vi "glyph_pass.vi"() -> (1 "image data":T1={"image type"=0, "image depth"=32, "image"=[0, 0, 0, 0, 0, 0, 0, 0, 0, 0, 0, 0, 0, 0, 0, 0, 0, 0, 0, 0, 255, 0, 0, 0, 255, 0, 0, 0, 255, 0, 0, 0, 255, 0, 0, 0, 255, 0, 0, 0, 0, 0, 0, 0, 0, 0, 0, 0, 0, 0, 0, 0, 0, 0, 0, 0, 0, 0, 0, 0, 0, 0, 0, 0, 0, 0, 0, 0, 0, 0, 0, 0, 0, 0, 0, 0, 255, 0, 0, 0, 255, 0, 0, 0, 255, 0, 255, 0, 255, 0, 255, 0, 255, 0, 255, 0, 255, 0, 255, 0, 255, 0, 255, 0, 255, 0, 0, 0, 255, 0, 0, 0, 0, 0, 0, 0, 0, 0, 0, 0, 0, 0, 0, 0, 0, 0, 0, 0, 0, 0, 0, 0, 0, 0, 0, 0, 255, 0, 0, 0, 255, 0, 255, 0, 255, 0, 255, 0, 255, 0, 128, 0, 255, 0, 128, 0, 255, 0, 128, 0, 255, 0, 128, 0, 255, 0, 128, 0, 255, 0, 128, 0, 255, 0, 128, 0, 255, 0, 0, 0, 0, 0, 0, 0, 0, 0, 0, 0, 0, 0, 0, 0, 0, 0, 0, 0, 255, 0, 0, 0, 255, 0, 255, 0, 255, 0, 128, 0, 255, 0, 128, 0, 255, 0, 128, 0, 255, 0, 128, 0, 255, 0, 128, 0, 255, 0, 128, 0, 255, 0, 128, 0, 255, 0, 128, 0, 255, 0, 128, 0, 255, 0, 128, 0, 255, 0, 0, 0, 0, 0, 0, 0, 0, 0, 0, 0, 0, 0, 0, 0, 255, 0, 0, 0, 255, 0, 255, 0, 255, 0, 128, 0, 255, 0, 128, 0, 255, 0, 128, 0, 255, 0, 128, 0, 255, 0, 128, 0, 255, 0, 128, 0, 255, 0, 128, 0, 255, 255, 255, 255, 255, 0, 128, 0, 255, 0, 128, 0, 255, 0, 0, 0, 0, 0, 0, 0, 0, 0, 0, 0, 255, 0, 0, 0, 255, 0, 255, 0, 255, 0, 128, 0, 255, 0, 128, 0, 255, 0, 128, 0, 255, 0, 128, 0, 255, 0, 128, 0, 255, 0, 128, 0, 255, 0, 128, 0, 255, 255, 255, 255, 255, 255, 255, 255, 255, 0, 128, 0, 255, 0, 128, 0, 255, 0, 128, 0, 255, 0, 0, 0, 0, 0, 0, 0, 255, 0, 0, 0, 255, 0, 255, 0, 255, 0, 128, 0, 255, 0, 128, 0, 255, 255, 255, 255, 255, 0, 128, 0, 255, 0, 128, 0, 255, 0, 128, 0, 255, 255, 255, 255, 255, 255, 255, 255, 255, 255, 255, 255, 255, 0, 128, 0, 255, 0, 128, 0, 255, 0, 128, 0, 255, 0, 0, 0, 255, 128, 128, 128, 255, 0, 0, 0, 255, 0, 255, 0, 255, 0, 128, 0, 255, 0, 128, 0, 255, 255, 255, 255, 255, 255, 255, 255, 255, 0, 128, 0, 255, 255, 255, 255, 255, 255, 255, 255, 255, 255, 255, 255, 255, 0, 128, 0, 255, 0, 128, 0, 255, 0, 128, 0, 255, 0, 128, 0, 255, 0, 0, 0, 255, 128, 128, 128, 255, 0, 0, 0, 255, 0, 255, 0, 255, 0, 128, 0, 255, 0, 128, 0, 255, 255, 255, 255, 255, 255, 255, 255, 255, 255, 255, 255, 255, 255, 255, 255, 255, 255, 255, 255, 255, 0, 128, 0, 255, 0, 128, 0, 255, 0, 128, 0, 255, 0, 128, 0, 255, 0, 128, 0, 255, 0, 0, 0, 255, 128, 128, 128, 255, 0, 0, 0, 255, 0, 255, 0, 255, 0, 128, 0, 255, 0, 128, 0, 255, 0, 128, 0, 255, 255, 255, 255, 255, 255, 255, 255, 255, 255, 255, 255, 255, 0, 128, 0, 255, 0, 128, 0, 255, 0, 128, 0, 255, 0, 128, 0, 255, 0, 128, 0, 255, 0, 128, 0, 255, 0, 0, 0, 255, 128, 128, 128, 0, 0, 0, 0, 255, 0, 0, 0, 255, 0, 255, 0, 255, 0, 128, 0, 255, 0, 128, 0, 255, 0, 128, 0, 255, 255, 255, 255, 255, 0, 128, 0, 255, 0, 128, 0, 255, 0, 128, 0, 255, 0, 128, 0, 255, 0, 128, 0, 255, 0, 128, 0, 255, 0, 0, 0, 255, 132, 132, 132, 255, 128, 128, 128, 0, 0, 0, 0, 255, 0, 0, 0, 255, 0, 255, 0, 255, 0, 128, 0, 255, 0, 128, 0, 255, 0, 128, 0, 255, 0, 128, 0, 255, 0, 128, 0, 255, 0, 128, 0, 255, 0, 128, 0, 255, 0, 128, 0, 255, 0, 128, 0, 255, 0, 128, 0, 255, 0, 0, 0, 255, 132, 132, 132, 255, 128, 128, 128, 0, 0, 0, 0, 0, 0, 0, 0, 255, 0, 0, 0, 255, 0, 128, 0, 255, 0, 128, 0, 255, 0, 128, 0, 255, 0, 128, 0, 255, 0, 128, 0, 255, 0, 128, 0, 255, 0, 128, 0, 255, 0, 128, 0, 255, 0, 128, 0, 255, 0, 0, 0, 255, 132, 132, 132, 255, 128, 128, 128, 0, 0, 0, 0, 0, 0, 0, 0, 0, 0, 0, 0, 0, 0, 0, 0, 255, 0, 0, 0, 255, 0, 0, 0, 255, 0, 128, 0, 255, 0, 128, 0, 255, 0, 128, 0, 255, 0, 128, 0, 255, 0, 128, 0, 255, 0, 0, 0, 255, 0, 0, 0, 255, 132, 132, 132, 255, 128, 128, 128, 0, 0, 0, 0, 0, 0, 0, 0, 0, 0, 0, 0, 0, 0, 0, 0, 0, 0, 0, 0, 0, 0, 0, 0, 0, 0, 0, 0, 255, 0, 0, 0, 255, 0, 0, 0, 255, 0, 0, 0, 255, 0, 0, 0, 255, 0, 0, 0, 255, 132, 132, 132, 255, 128, 128, 128, 255, 128, 128, 128, 0, 0, 0, 0, 0, 0, 0, 0, 0, 0, 0, 0, 0, 0, 0, 0, 0, 0, 0, 0, 0, 0, 0, 0, 0, 0, 0, 0, 0, 0, 0, 0, 0, 0, 0, 0, 255, 128, 128, 128, 255, 128, 128, 128, 255, 128, 128, 128, 255, 128, 128, 128, 255, 128, 128, 128, 0, 0, 0, 0, 0, 0, 0, 0, 0, 0, 0, 0, 0, 0, 0, 0, 0, 0, 0, 0], "mask"=[7, 192, 31, 240, 63, 248, 127, 252, 127, 252, 255, 254, 255, 255, 255, 255, 255, 255, 255, 255, 127, 255, 127, 255, 63, 254, 31, 252, 7, 248, 3, 224], "colors"=[], "Rectangle"={"left"=0, "top"=0, "right"=16, "bottom"=16}})   [LabVIEW 2015]
uses:
  <vilib>/picture/picture.llb/imagedata.ctl
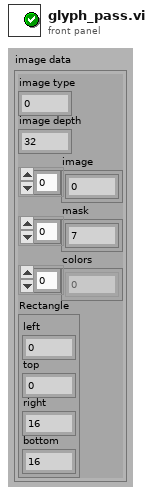
[diagram p1: front panel]
types:
  T1 = typedef "imagedata.ctl" = cluster{"image type":i32, "image depth":i32, "image":u8[], "mask":u8[], "colors":u32[], "Rectangle":cluster{"left":i16, "top":i16, "right":i16, "bottom":i16}}
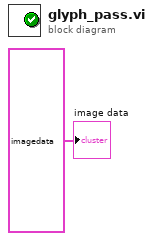
[diagram p0: block diagram]
diagram:
  "image data" <- T1 {"image type"=0, "image depth"=32, "image"=[0, 0, 0, 0, 0, 0, 0, 0, 0, 0, 0, 0, 0, 0, 0, 0, 0, 0, 0, 0, 255, 0, 0, 0, 255, 0, 0, 0, 255, 0, 0, 0, 255, 0, 0, 0, 255, 0, 0, 0, 0, 0, 0, 0, 0, 0, 0, 0, 0, 0, 0, 0, 0, 0, 0, 0, 0, 0, 0, 0, 0, 0, 0, 0, 0, 0, 0, 0, 0, 0, 0, 0, 0, 0, 0, 0, 255, 0, 0, 0, 255, 0, 0, 0, 255, 0, 255, 0, 255, 0, 255, 0, 255, 0, 255, 0, 255, 0, 255, 0, 255, 0, 255, 0, 255, 0, 0, 0, 255, 0, 0, 0, 0, 0, 0, 0, 0, 0, 0, 0, 0, 0, 0, 0, 0, 0, 0, 0, 0, 0, 0, 0, 0, 0, 0, 0, 255, 0, 0, 0, 255, 0, 255, 0, 255, 0, 255, 0, 255, 0, 128, 0, 255, 0, 128, 0, 255, 0, 128, 0, 255, 0, 128, 0, 255, 0, 128, 0, 255, 0, 128, 0, 255, 0, 128, 0, 255, 0, 0, 0, 0, 0, 0, 0, 0, 0, 0, 0, 0, 0, 0, 0, 0, 0, 0, 0, 255, 0, 0, 0, 255, 0, 255, 0, 255, 0, 128, 0, 255, 0, 128, 0, 255, 0, 128, 0, 255, 0, 128, 0, 255, 0, 128, 0, 255, 0, 128, 0, 255, 0, 128, 0, 255, 0, 128, 0, 255, 0, 128, 0, 255, 0, 128, 0, 255, 0, 0, 0, 0, 0, 0, 0, 0, 0, 0, 0, 0, 0, 0, 0, 255, 0, 0, 0, 255, 0, 255, 0, 255, 0, 128, 0, 255, 0, 128, 0, 255, 0, 128, 0, 255, 0, 128, 0, 255, 0, 128, 0, 255, 0, 128, 0, 255, 0, 128, 0, 255, 255, 255, 255, 255, 0, 128, 0, 255, 0, 128, 0, 255, 0, 0, 0, 0, 0, 0, 0, 0, 0, 0, 0, 255, 0, 0, 0, 255, 0, 255, 0, 255, 0, 128, 0, 255, 0, 128, 0, 255, 0, 128, 0, 255, 0, 128, 0, 255, 0, 128, 0, 255, 0, 128, 0, 255, 0, 128, 0, 255, 255, 255, 255, 255, 255, 255, 255, 255, 0, 128, 0, 255, 0, 128, 0, 255, 0, 128, 0, 255, 0, 0, 0, 0, 0, 0, 0, 255, 0, 0, 0, 255, 0, 255, 0, 255, 0, 128, 0, 255, 0, 128, 0, 255, 255, 255, 255, 255, 0, 128, 0, 255, 0, 128, 0, 255, 0, 128, 0, 255, 255, 255, 255, 255, 255, 255, 255, 255, 255, 255, 255, 255, 0, 128, 0, 255, 0, 128, 0, 255, 0, 128, 0, 255, 0, 0, 0, 255, 128, 128, 128, 255, 0, 0, 0, 255, 0, 255, 0, 255, 0, 128, 0, 255, 0, 128, 0, 255, 255, 255, 255, 255, 255, 255, 255, 255, 0, 128, 0, 255, 255, 255, 255, 255, 255, 255, 255, 255, 255, 255, 255, 255, 0, 128, 0, 255, 0, 128, 0, 255, 0, 128, 0, 255, 0, 128, 0, 255, 0, 0, 0, 255, 128, 128, 128, 255, 0, 0, 0, 255, 0, 255, 0, 255, 0, 128, 0, 255, 0, 128, 0, 255, 255, 255, 255, 255, 255, 255, 255, 255, 255, 255, 255, 255, 255, 255, 255, 255, 255, 255, 255, 255, 0, 128, 0, 255, 0, 128, 0, 255, 0, 128, 0, 255, 0, 128, 0, 255, 0, 128, 0, 255, 0, 0, 0, 255, 128, 128, 128, 255, 0, 0, 0, 255, 0, 255, 0, 255, 0, 128, 0, 255, 0, 128, 0, 255, 0, 128, 0, 255, 255, 255, 255, 255, 255, 255, 255, 255, 255, 255, 255, 255, 0, 128, 0, 255, 0, 128, 0, 255, 0, 128, 0, 255, 0, 128, 0, 255, 0, 128, 0, 255, 0, 128, 0, 255, 0, 0, 0, 255, 128, 128, 128, 0, 0, 0, 0, 255, 0, 0, 0, 255, 0, 255, 0, 255, 0, 128, 0, 255, 0, 128, 0, 255, 0, 128, 0, 255, 255, 255, 255, 255, 0, 128, 0, 255, 0, 128, 0, 255, 0, 128, 0, 255, 0, 128, 0, 255, 0, 128, 0, 255, 0, 128, 0, 255, 0, 0, 0, 255, 132, 132, 132, 255, 128, 128, 128, 0, 0, 0, 0, 255, 0, 0, 0, 255, 0, 255, 0, 255, 0, 128, 0, 255, 0, 128, 0, 255, 0, 128, 0, 255, 0, 128, 0, 255, 0, 128, 0, 255, 0, 128, 0, 255, 0, 128, 0, 255, 0, 128, 0, 255, 0, 128, 0, 255, 0, 128, 0, 255, 0, 0, 0, 255, 132, 132, 132, 255, 128, 128, 128, 0, 0, 0, 0, 0, 0, 0, 0, 255, 0, 0, 0, 255, 0, 128, 0, 255, 0, 128, 0, 255, 0, 128, 0, 255, 0, 128, 0, 255, 0, 128, 0, 255, 0, 128, 0, 255, 0, 128, 0, 255, 0, 128, 0, 255, 0, 128, 0, 255, 0, 0, 0, 255, 132, 132, 132, 255, 128, 128, 128, 0, 0, 0, 0, 0, 0, 0, 0, 0, 0, 0, 0, 0, 0, 0, 0, 255, 0, 0, 0, 255, 0, 0, 0, 255, 0, 128, 0, 255, 0, 128, 0, 255, 0, 128, 0, 255, 0, 128, 0, 255, 0, 128, 0, 255, 0, 0, 0, 255, 0, 0, 0, 255, 132, 132, 132, 255, 128, 128, 128, 0, 0, 0, 0, 0, 0, 0, 0, 0, 0, 0, 0, 0, 0, 0, 0, 0, 0, 0, 0, 0, 0, 0, 0, 0, 0, 0, 0, 255, 0, 0, 0, 255, 0, 0, 0, 255, 0, 0, 0, 255, 0, 0, 0, 255, 0, 0, 0, 255, 132, 132, 132, 255, 128, 128, 128, 255, 128, 128, 128, 0, 0, 0, 0, 0, 0, 0, 0, 0, 0, 0, 0, 0, 0, 0, 0, 0, 0, 0, 0, 0, 0, 0, 0, 0, 0, 0, 0, 0, 0, 0, 0, 0, 0, 0, 0, 255, 128, 128, 128, 255, 128, 128, 128, 255, 128, 128, 128, 255, 128, 128, 128, 255, 128, 128, 128, 0, 0, 0, 0, 0, 0, 0, 0, 0, 0, 0, 0, 0, 0, 0, 0, 0, 0, 0, 0], "mask"=[7, 192, 31, 240, 63, 248, 127, 252, 127, 252, 255, 254, 255, 255, 255, 255, 255, 255, 255, 255, 127, 255, 127, 255, 63, 254, 31, 252, 7, 248, 3, 224], "colors"=[], "Rectangle"={"left"=0, "top"=0, "right"=16, "bottom"=16}} ("image data")
